vi "ArduinoSerialTest2.vi"() -> ()   [LabVIEW 2013]
uses:
  <vilib>/Instr/_visa.llb/VISA Set IO Buffer Mask.ctl
  <vilib>/Instr/_visa.llb/VISA Configure Serial Port (Instr).vi
panel:
  in  "-90":bool
  in  "-270":bool
  in  "-180":bool
  in  "-360":bool
  in  "+360":bool
  in  "Auto":dbl
  in  "+180":bool
  in  "+270":bool
  in  "+90":bool
  in  "Manual":dbl
  in  "stop":bool
  in  "Go":bool
  in  "VISA resource name":refnum<visa-resource-name>
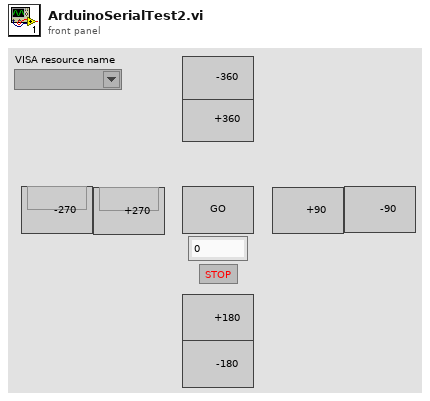
[diagram p1: front panel]
types:
  T1 = typedef "VISA Set IO Buffer Mask.ctl" = u16
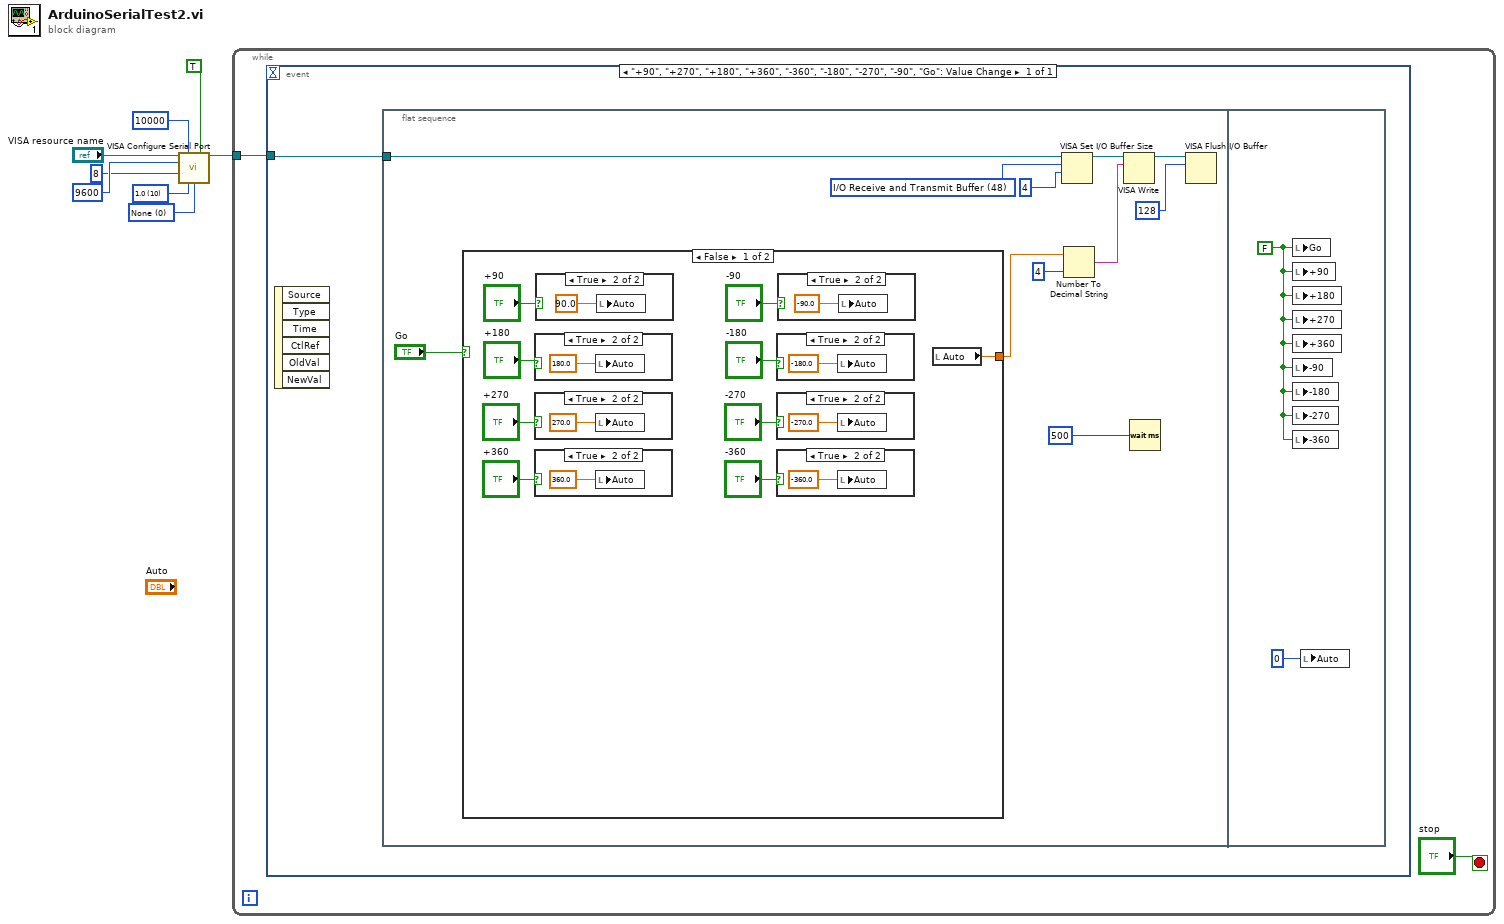
[diagram p0: block diagram]
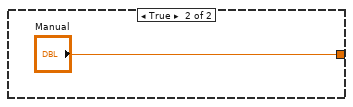
[diagram p10: hidden frame]
diagram:
  w3 = u16 0 items=["None", "XON/XOFF", "RTS/CTS", "XON/XOFF & RTS/CTS", "DTR/DSR", "XON/XOFF & DTR/DSR"] ("flow control (0:none)")
  w4 = u16 10 items=["1.0"=10, "1.5"=15, "2.0"=20] ("stop bits (10: 1 bit)")
  n1 = call-poly "VISA Configure Serial Port"("VISA resource name"="VISA resource name", "timeout (10sec)"=u32 10000, "Enable Termination\nChar (T)"=TRUE ("Enable Termination\nChar (T)"), "baud rate (9600)"=u32 9600, "data bits (8)"=u16 8, "stop bits (10: 1 bit)"=w4, "flow control (0:none)"=w3) -> ("VISA resource name out"=w8:refnum<visa-resource-name>)  [unwired: 7 in, 1 out]
  n2 = while {
    tunnel: w8 -> [w10]
    stop <- "stop" stop-if-true
    n3 = event shown="[0] \"+90\", \"+270\", \"+180\", \"+360\", \"-360\", \"-180\", \"-270\", \"-90\", \"Go\": Value Change" {
      selector: _ -> [_]
      dyn-events: _ -> [_]
      timeout: _ -> [_]
      tunnel: w10 -> [w11]
      event "+90", "+270", "+180", "+360", "-360", "-180", "-270", "-90", "Go": Value Change {
        n4 = event-data() -> ()  [unwired: 1 in, 6 out]
        n5 = flat-sequence {
          tunnel: w11 -> [w22]
          frame #0 {
            w17 = T1 48 items=["I/O Receive Buffer"=16, "I/O Transmit Buffer"=32, "I/O Receive and Transmit Buffer"=48] ("Mask")
            n6 = case shown="False" "Go" {
              tunnel: [w28 "Manual"] -> w15
              frame False {
                n7 = case shown="True" "+180" {
                  frame False {
                  }
                  frame True {
                    n8 = local write "Auto"(180.0 ("Numeric")) -> ()
                  }
                }
                n9 = case shown="True" "+270" {
                  frame False {
                  }
                  frame True {
                    n10 = local write "Auto"(270.0 ("Numeric")) -> ()
                  }
                }
                n11 = case shown="True" "+360" {
                  frame False {
                  }
                  frame True {
                    n12 = local write "Auto"(360.0 ("Numeric")) -> ()
                  }
                }
                n13 = case shown="True" "+90" {
                  frame False {
                  }
                  frame True {
                    n14 = local write "Auto"(90.0 ("Numeric")) -> ()
                  }
                }
                n15 = case shown="True" "-180" {
                  frame False {
                  }
                  frame True {
                    n16 = local write "Auto"(-180.0 ("Numeric")) -> ()
                  }
                }
                n17 = case shown="True" "-270" {
                  frame False {
                  }
                  frame True {
                    n18 = local write "Auto"(-270.0 ("Numeric")) -> ()
                  }
                }
                n19 = case shown="True" "-360" {
                  frame False {
                  }
                  frame True {
                    n20 = local write "Auto"(-360.0 ("Numeric")) -> ()
                  }
                }
                n21 = case shown="True" "-90" {
                  frame False {
                  }
                  frame True {
                    n22 = local write "Auto"(-90.0 ("Numeric")) -> ()
                  }
                }
                n23 = local read "Auto"() -> (w28:dbl)
              }
              frame True {
              }
            }
            n24 = VISA Set I/O Buffer Size(VISA resource name=w22, mask (16)=w17, size (4096)=u32 4) -> (VISA resource name out=w20:refnum<visa-resource-name>)  [unwired: 1 in, 1 out]
            n25 = Number To Decimal String(number=w15, width (-)=4) -> (decimal integer string=w14:string)
            n26 = VISA Write(VISA resource name=w20, write buffer=w14) -> (VISA resource name out=w18:refnum<visa-resource-name>)  [unwired: 1 in, 2 out]
            n27 = Wait (ms)(milliseconds to wait=u32 500) -> ()  [unwired: 1 out]
            n28 = VISA Flush I/O Buffer(VISA resource name=w18, mask (16)=128) -> ()  [unwired: 1 in, 2 out]
          }
          frame #1 {
            w41 = FALSE
            n29 = local write "Go"(w41) -> ()
            n30 = local write "+90"(w41) -> ()
            n31 = local write "+180"(w41) -> ()
            n32 = local write "+270"(w41) -> ()
            n33 = local write "+360"(w41) -> ()
            n34 = local write "-90"(w41) -> ()
            n35 = local write "-180"(w41) -> ()
            n36 = local write "-270"(w41) -> ()
            n37 = local write "-360"(w41) -> ()
            n38 = local write "Auto"(0) -> ()
          }
        }
      }
    }
  }
